vi "Data.vi"(8 "error in (no error)":errorcluster, 11 "PB Msg Template in":refnum<class "Msg.lvclass">) -> (0 "error out":errorcluster, 2 "Data":T1, 3 "PB Msg Template out":refnum<class "Msg.lvclass">)   [LabVIEW 2020, in "Events.lvlib" / "Msg.lvclass"]
uses:
  Msg.lvclass
  Data.ctl
  Event/Data.ctl
  EventLevel/Enumeration.ctl
  Error/Data.ctl
  Msg.lvclass/Msg.ctl
  Events.lvlib
  Error/Error.lvlib
  EventLevel/EventLevel.lvlib
  Event/Event.lvlib
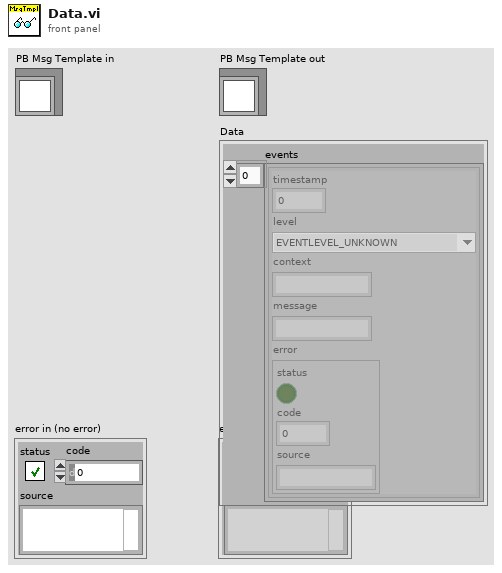
[diagram p1: front panel]
types:
  T1 = typedef "Events.lvlib/Data.ctl" = cluster{"events":T2[]}
  T2 = typedef "Event.lvlib/Data.ctl" = cluster{"timestamp":i64, "level":T3, "context":string, "message":string, "error":T4}
  T3 = typedef "EventLevel.lvlib/Enumeration.ctl" = enum16{"EVENTLEVEL_UNKNOWN", "EVENTLEVEL_DEBUG", "EVENTLEVEL_INFO", "EVENTLEVEL_WARNING", "EVENTLEVEL_ERROR"}
  T4 = typedef "Error.lvlib/Data.ctl" = errorcluster
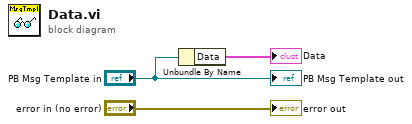
[diagram p0: block diagram]
diagram:
  n1 = Unbundle By Name("PB Msg Template in") -> ("Data"=→"Data":T1)
  "error out" <- "error in (no error)"
  "PB Msg Template out" <- "PB Msg Template in"
